vi "Build All Class HTML Documentation.vi"(6 "Requirement":string="Labstache", 7 "Destination":path=path "", 8 "Error In":errorcluster, 11 "Source In":path=path "") -> (0 "Error Out":errorcluster, 3 "Source Out":path)   [LabVIEW 2018, in "Scripts.lvlib"]
uses:
  Scripts.lvlib
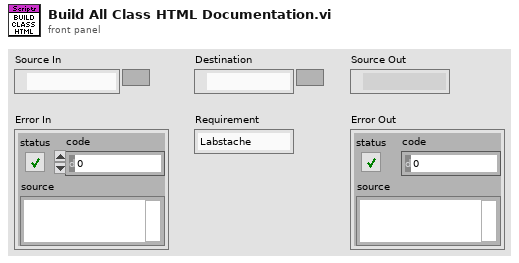
[diagram p1: front panel]
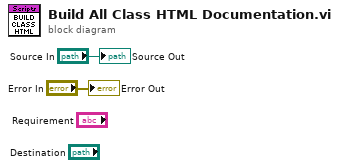
[diagram p0: block diagram]
diagram:
  "Error Out" <- "Error In"
  "Source Out" <- "Source In"
